vi "LoadCalibrationFile.vi"(8 "error in (no error)":errorcluster, 11 "Path":path) -> (0 "error out":errorcluster, 3 "CalibrationState":T1)   [LabVIEW 2013]
panel:
  # "CalibrationDone"
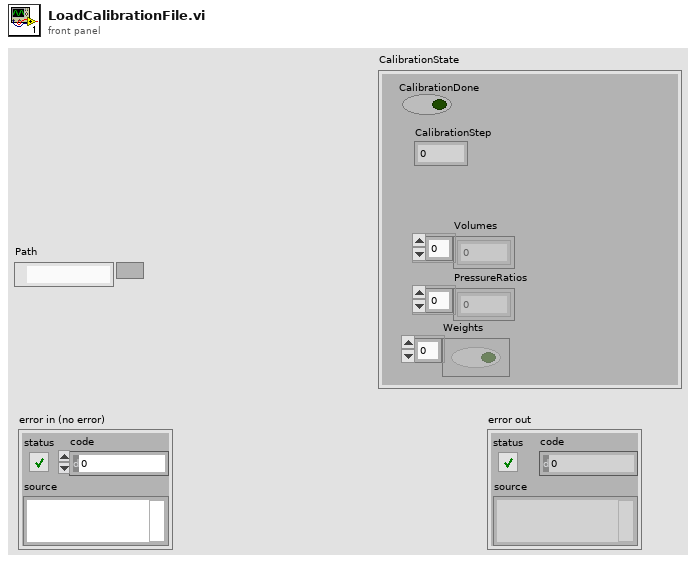
[diagram p1: front panel]
types:
  T1 = cluster{bool, "CalibrationStep":u32, "Volumes":dbl[], "PressureRatios":dbl[], "Weights":bool[]}
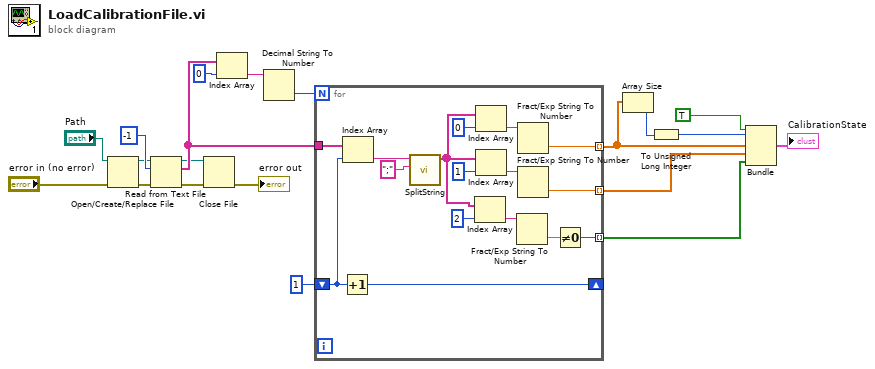
[diagram p0: block diagram]
diagram:
  n1 = Open/Create/Replace File(file path (use dialog)="Path", error in="error in (no error)") -> (refnum out=w15:refnum<file>, error out=w16:errorcluster)  [unwired: 4 in, 1 out]
  n2 = Read from Text File(file (use dialog)=w15, count=-1, error in=w16) -> (refnum out=w6:refnum<file>, text=w10:string[], error out=w5:errorcluster)  [unwired: 1 in, 1 out]
  n3 = Close File(refnum=w6, error in=w5) -> (error out=→"error out":errorcluster)  [unwired: 1 out]
  n4 = Index Array(array=w10, index=0) -> (element=w11:string)
  n5 = Decimal String To Number(string=w11) -> (number=w14:i32)  [unwired: 2 in, 1 out]
  n6 = for {
    N: w14 -> [_]
    shift-right: [w36] -> _
    shift-left: 1 -> [w32]
    tunnel: w10 -> [w35]
    tunnel: [w27] -> w4 mode=indexing
    tunnel: [w26] -> w9 mode=indexing
    tunnel: [w21] -> w1 mode=indexing
    n7 = Increment(x=w32) -> (x+1=w36:i32)
    n8 = Index Array(array=w35, index=w32) -> (element=w34:string)
    n9 = call "SplitString.vi"("Separator"=";", "String[in]"=w34) -> ("Slices"=w23:string[])  [unwired: 9 in]
    n10 = Index Array(array=w23, index=2) -> (element=w25:string)
    n11 = Index Array(array=w23, index=0) -> (element=w29:string)
    n12 = Index Array(array=w23, index=1) -> (element=w28:string)
    n13 = Fract/Exp String To Number(string=w25) -> (number=w22:dbl)  [unwired: 3 in, 1 out]
    n14 = Fract/Exp String To Number(string=w29) -> (number=w27:dbl)  [unwired: 3 in, 1 out]
    n15 = Fract/Exp String To Number(string=w28) -> (number=w26:dbl)  [unwired: 3 in, 1 out]
    n16 = Not Equal To 0?(x=w22) -> (x != 0?=w21:bool)
  }
  n17 = Array Size(array=w4) -> (size(s)=w2:i32)
  n18 = To Unsigned Long Integer(number=w2) -> (unsigned 32bit integer=w3:u32)
  n19 = Bundle(TRUE, w3, w4, w9, w1) -> (→"CalibrationState":cluster{bool, u32, dbl[], dbl[], bool[]})  [unwired: 1 in]
